vi "pid.vi"() -> (0 "Direct M3":bool, 1 "Pwm M3":dbl format="%#_13g", 2 "Pwm M2":dbl format="%#_13g", 3 "Pwm M1":dbl format="%#_13g", 4 "Direct M2":bool, 6 "Direct M1":bool, 9 "Counter Value 3":i32, 10 "Counter Value 2":i32, 11 "Counter Value":i32)   [LabVIEW 2015]
uses:
  <vilib>/myRIO/Common/Instrument Driver Framework/myRIO v1.0/Encoder/typedefs/Encoder Signal Mode.ctl
  <vilib>/myRIO/Instrument Drivers/Onboard IO/Encoder/typedefs/Encoder Reference.ctl
  <vilib>/myRIO/Common/Instrument Driver Framework/Utilities/typedefs/myRIO Generic Hardware Reference.ctl
  <vilib>/myRIO/Common/Instrument Driver Framework/Utilities/typedefs/Hardware Version Enum.ctl
  <vilib>/myRIO/Common/Instrument Driver Framework/Utilities/typedefs/myRIO v1.0 Reference.ctl
  <vilib>/myRIO/Common/Instrument Driver Framework/Utilities/typedefs/Generic FPGA Reference.ctl
  <vilib>/myRIO/Common/Instrument Driver Framework/myRIO v1.0/Encoder/typedefs/Encoder Channels Enum.ctl
  <vilib>/myRIO/Common/Instrument Driver Framework/myRIO v1.0/Encoder/typedefs/Encoder Configuration v1.0.ctl
  <vilib>/userdefined/High Color/nirio_resource_hc.ctl
  <vilib>/myRIO/Instrument Drivers/Onboard IO/DIO/typedefs/DIO Reference.ctl
  <vilib>/myRIO/Common/Instrument Driver Framework/myRIO v1.0/DIO/typedefs/DIO Channels List.ctl
  <vilib>/myRIO/Common/Instrument Driver Framework/myRIO v1.0/DIO/typedefs/DIO Channels Enum.ctl
  <vilib>/myRIO/Instrument Drivers/Onboard IO/PWM/typedefs/PWM Reference.ctl
  <vilib>/myRIO/Common/Instrument Driver Framework/myRIO v1.0/PWM/typedefs/PWM Channels Enum.ctl
  <vilib>/myRIO/Instrument Drivers/Onboard IO/PWM/typedefs/PWM Configuration.ctl
  <vilib>/myRIO/Common/Instrument Driver Framework/Utilities/vis/Is FPGA Ref Available.vi
  <vilib>/myRIO/Common/Instrument Driver Framework/myRIO v1.0/Encoder/vis/myRIO v1.1 Open Encoder.vi
  <vilib>/myRIO/Instrument Drivers/Onboard IO/Encoder/vis/Read.vi
  <vilib>/myRIO/Common/Instrument Driver Framework/myRIO v1.0/DIO/vis/myRIO v1.1 Open DIO.vi
  <vilib>/myRIO/Instrument Drivers/Onboard IO/DIO/vis/Write.vi
  <vilib>/myRIO/Common/Instrument Driver Framework/myRIO v1.0/PWM/vis/myRIO v1.1 Open PWM.vi
  <vilib>/myRIO/Instrument Drivers/Onboard IO/PWM/vis/Set Duty Cycle and Frequency.vi
  <vilib>/myRIO/Common/Instrument Driver Framework/Utilities/vis/Validate Channels.vi
  <vilib>/myRIO/Common/Instrument Driver Framework/myRIO v1.0/Encoder/vis/myRIO v1.0 Reserve Encoder.vi
  <vilib>/myRIO/Common/Instrument Driver Framework/myRIO v1.0/DIO/vis/myRIO v1.0 Reserve DIO.vi
  <vilib>/myRIO/Common/Instrument Driver Framework/myRIO v1.0/PWM/vis/myRIO v1.0 Reserve PWM.vi
  <vilib>/myRIO/Common/Instrument Driver Framework/myRIO v1.0/Encoder/vis/myRIO v1.0 Build MUX Configuration Encoder.vi
  <vilib>/myRIO/Common/Instrument Driver Framework/myRIO v1.0/Resource Manager/vis/myRIO v1.0 Reserve Channel List.vi
  <vilib>/myRIO/Common/Instrument Driver Framework/myRIO v1.0/DIO/vis/myRIO v1.0 Build MUX Configuration DIO.vi
  <vilib>/myRIO/Common/Instrument Driver Framework/myRIO v1.0/PWM/vis/myRIO v1.0 Build MUX Configuration PWM.vi
  <vilib>/myRIO/Common/Instrument Driver Framework/myRIO v1.0/Resource Manager/vis/myRIO v1.0 Create Configuration List.vi
  <vilib>/myRIO/Common/Instrument Driver Framework/myRIO v1.0/Resource Manager/vis/myRIO v1.0 Reserve Channel.vi
  <vilib>/myRIO/Common/Instrument Driver Framework/myRIO v1.0/Resource Manager/vis/myRIO v1.0 Unreserve Channel.vi
  <vilib>/myRIO/Common/Instrument Driver Framework/myRIO v1.0/Resource Manager/vis/myRIO v1.0 Build Mutex Name.vi
  <vilib>/Utility/VariantDataType/GetNumericInfo.vi
  <vilib>/Utility/error.llb/Error Cluster From Error Code.vi
  <vilib>/myRIO/Common/Instrument Driver Framework/myRIO v1.0/myRIO v1.1 Open.vi
  <vilib>/myRIO/Common/Instrument Driver Framework/Utilities/vis/IO Manager.vi
  <vilib>/myRIO/Common/Instrument Driver Framework/Utilities/vis/Configuration Manager.vi
  <vilib>/myRIO/Common/Instrument Driver Framework/myRIO v1.0/Resource Manager/vis/myRIO v1.0 Configure IO.vi
  <vilib>/myRIO/Common/Instrument Driver Framework/myRIO v1.0/myRIO v1.0 Close.vi
  <vilib>/myRIO/Common/Instrument Driver Framework/myRIO v1.0/Encoder/vis/myRIO v1.0 Configure Encoder.vi
  <vilib>/myRIO/Common/Instrument Driver Framework/myRIO v1.0/Encoder/vis/myRIO v1.0 Read Encoder.vi
  <vilib>/addons/control/pid/pid.llb/PID (DBL).vi
  <vilib>/myRIO/Common/Instrument Driver Framework/myRIO v1.0/DIO/vis/myRIO v1.0 Write DIO.vi
  <vilib>/myRIO/Common/Instrument Driver Framework/myRIO v1.0/PWM/vis/myRIO v1.0 Write PWM.vi
  <vilib>/myRIO/Express VI/Onboard IO/Encoder/Encoder Express VI.xnode
  <vilib>/myRIO/Instrument Drivers/Onboard IO/Encoder/vis/myRIO Encoder Open.xnode
  <vilib>/myRIO/Common/Instrument Driver Framework/myRIO v1.0/Encoder/typedefs/Encoder Count Direction Enum.ctl
  <vilib>/myRIO/Express VI/Onboard IO/DO/DO Express VI.xnode
  <vilib>/myRIO/Instrument Drivers/Onboard IO/DIO/vis/myRIO DIO Open.xnode
  <vilib>/myRIO/Express VI/Onboard IO/PWM/PWM Express VI.xnode
  <vilib>/myRIO/Instrument Drivers/Onboard IO/PWM/vis/myRIO PWM Open.xnode
  <vilib>/myRIO/Instrument Drivers/Onboard IO/Encoder/Encoder.lvlib
  <vilib>/addons/control/pid/NI_PID_pid.lvlib
  <vilib>/myRIO/Instrument Drivers/Onboard IO/DIO/DIO.lvlib
  <vilib>/myRIO/Instrument Drivers/Onboard IO/PWM/PWM.lvlib
panel:
  out "Waveform Chart 3":dynamicdata(graph)
  in  "PID gains 3":T1={"proportional gain (Kc)"=2.0, "integral time (Ti, min)"=0.001, "derivative time (Td, min)"=0.0} {"derivative time (Td, min)" format="%.3f"; "integral time (Ti, min)" format="%.3f"; "proportional gain (Kc)" format="%.3f"}
  out "output 3":dbl format="%.2f"
  in  "rpm 6":dbl(slide) scale=-230.0..230.0
  out "rpm 5":dbl
  out "Omega2 (rad/s) 3":dbl
  out "Omega(c/s) 3":dbl
  in  "Reset Counter 3":bool
  out "Waveform Chart 2":dynamicdata(graph)
  in  "PID gains 2":T1={"proportional gain (Kc)"=2.0, "integral time (Ti, min)"=0.001, "derivative time (Td, min)"=0.0} {"derivative time (Td, min)" format="%.3f"; "integral time (Ti, min)" format="%.3f"; "proportional gain (Kc)" format="%.3f"}
  out "output 2":dbl format="%.2f"
  in  "rpm 4":dbl(slide) scale=-230.0..230.0
  out "rpm 3":dbl
  out "Omega2 (rad/s) 2":dbl
  out "Omega(c/s) 2":dbl
  in  "Reset Counter 2":bool
  in  "stop":bool
  in  "Reset Counter":bool
  out "Omega(c/s)":dbl
  out "Omega2 (rad/s)":dbl
  out "rpm 2":dbl
  in  "rpm":dbl(slide) scale=-230.0..230.0
  out "output":dbl format="%.2f"
  in  "PID gains":T1={"proportional gain (Kc)"=2.0, "integral time (Ti, min)"=0.001, "derivative time (Td, min)"=0.0} {"derivative time (Td, min)" format="%.3f"; "integral time (Ti, min)" format="%.3f"; "proportional gain (Kc)" format="%.3f"}
  out "Waveform Chart":dynamicdata(graph)
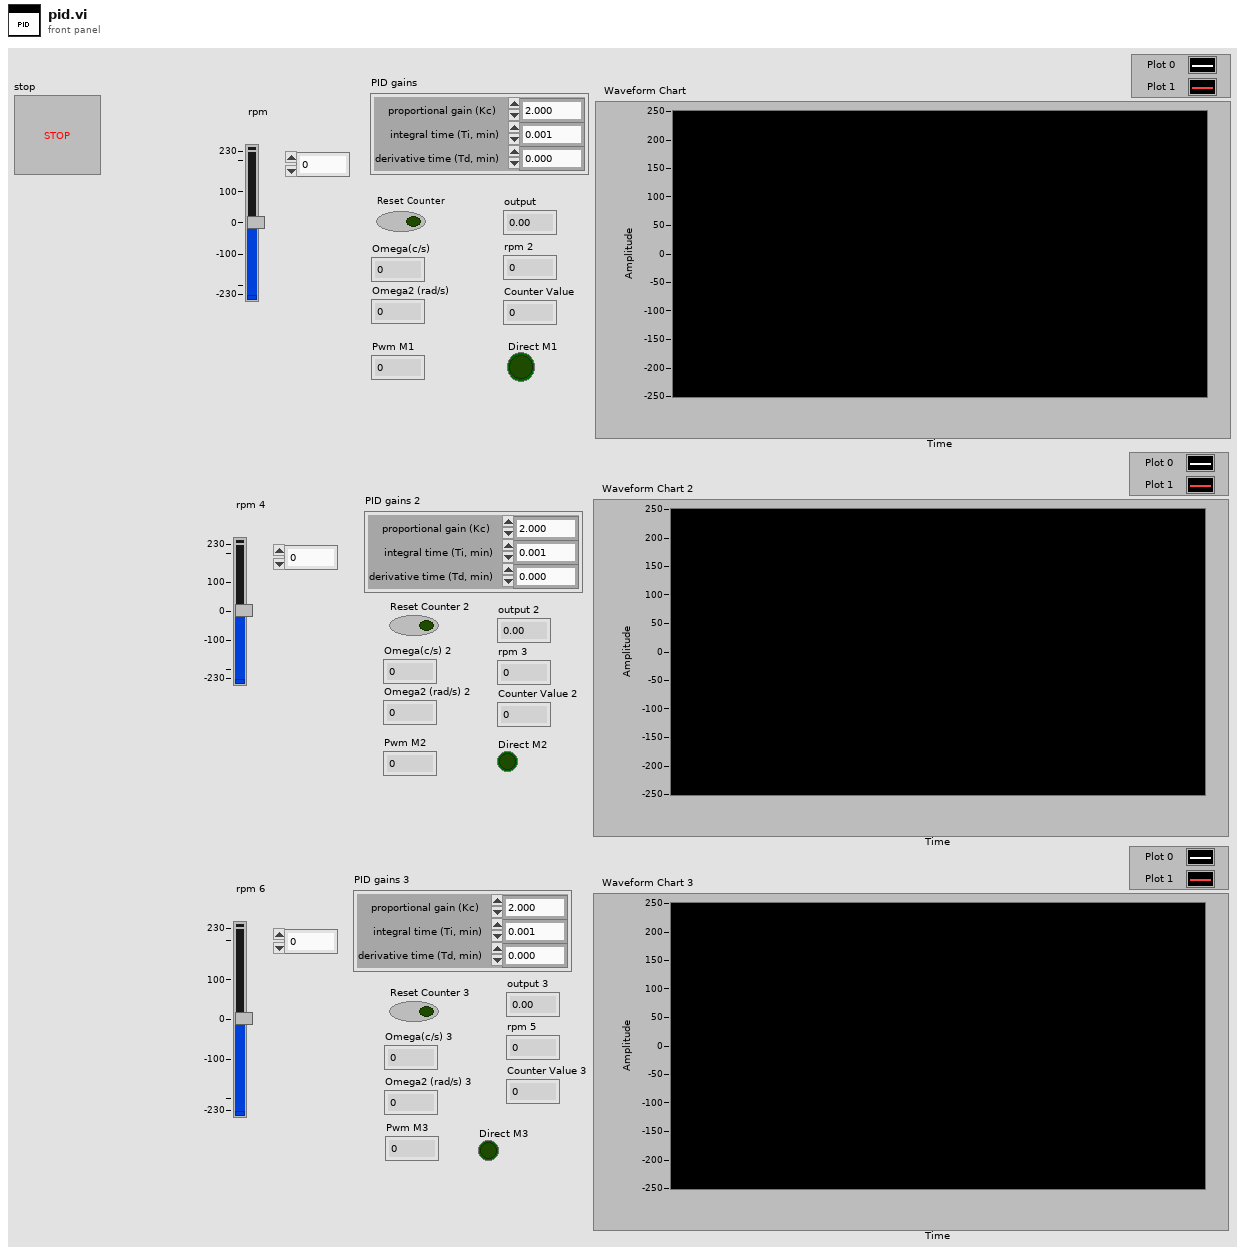
[diagram p1: front panel]
types:
  T1 = cluster{"proportional gain (Kc)":dbl, "integral time (Ti, min)":dbl, "derivative time (Td, min)":dbl}
  T2 = typedef "Encoder.lvlib/Encoder Reference.ctl" = cluster{"myRIO Reference":T3, "Encoder Channels Enum":T7}
  T3 = typedef "myRIO Generic Hardware Reference.ctl" = cluster{"myRIO Model":T4, "myRIO Hardware Reference":T5}
  T4 = typedef "Hardware Version Enum.ctl" = enum16{"Unknown", "myRIO-1900", "myRIO-1950", "roboRIO"}
  T5 = typedef "myRIO v1.0 Reference.ctl" = cluster{"Generic FPGA Reference":T6, "Allow multiple opens":bool}
  T6 = typedef "Generic FPGA Reference.ctl" = refnum<k20>
  T7 = typedef "Encoder Channels Enum.ctl" = enum16{"Not Connected", "C/ENC0", "C/ENC1", "A/ENC", "B/ENC", "DIO/ENC0", "DIO/ENC1", "DIO/ENC2", "DIO/ENC3", "DIO/ENC4"}
  T8 = typedef "Encoder Signal Mode.ctl" = enum16{"Quadrature phase signal", "Step and direction signal"}
  T9 = typedef "nirio_resource_hc.ctl" = tag
  T10 = typedef "PWM.lvlib/PWM Reference.ctl" = cluster{"myRIO Reference":T3, "PWM Channels Enum":T11, "PWM Configuration":T12}
  T11 = typedef "PWM Channels Enum.ctl" = enum16{"Not Connected", "C/PWM0", "C/PWM1", "A/PWM0", "A/PWM1", "A/PWM2", "B/PWM0", "B/PWM1", "B/PWM2", "PWM/PWM0", "PWM/PWM1", "PWM/PWM2", "PWM/PWM3", "PWM/PWM4", "PWM/PWM5", "PWM/PWM6", "PWM/PWM7", "PWM/PWM8", "PWM/PWM9"}
  T12 = typedef "PWM.lvlib/PWM Configuration.ctl" = cluster{"Frequency":dbl, "Duty Cycle":dbl}
  T13 = typedef "DIO.lvlib/DIO Reference.ctl" = cluster{"myRIO Reference":T3, "DIO Channels List":T14}
  T14 = typedef "DIO Channels List.ctl" = T15[]
  T15 = typedef "DIO Channels Enum.ctl" = enum16{"Not Connected", "C/DIO0", "C/DIO1", "C/DIO2", "C/DIO3", "C/DIO4", "C/DIO5", "C/DIO6", "C/DIO7", "A/DIO0", "A/DIO1", "A/DIO2", "A/DIO3", "A/DIO4", "A/DIO5", "A/DIO6", "A/DIO7", "A/DIO8", "A/DIO9", "A/DIO10", "A/DIO11", "A/DIO12", "A/DIO13", "A/DIO14", "A/DIO15", "B/DIO0", "B/DIO1", "B/DIO2", "B/DIO3", "B/DIO4", "B/DIO5", "B/DIO6", "B/DIO7", "B/DIO8", "B/DIO9", "B/DIO10", "B/DIO11", "B/DIO12", "B/DIO13", "B/DIO14", "B/DIO15", "LED0", "LED1", "LED2", "LED3", "Button0", "DIO/DIO0", "DIO/DIO1", "DIO/DIO2", "DIO/DIO3", "DIO/DIO4", "DIO/DIO5", "DIO/DIO6", "DIO/DIO7", "DIO/DIO8", "DIO/DIO9", "SPI/CS0", "SPI/CS1", "SPI/CS2", "SPI/CS3", "LED RADIO (Green)", "LED RADIO (Red)", "LED COMM (Green)", "LED COMM (Red)", "LED MODE (Green)", "LED MODE (Red)"}
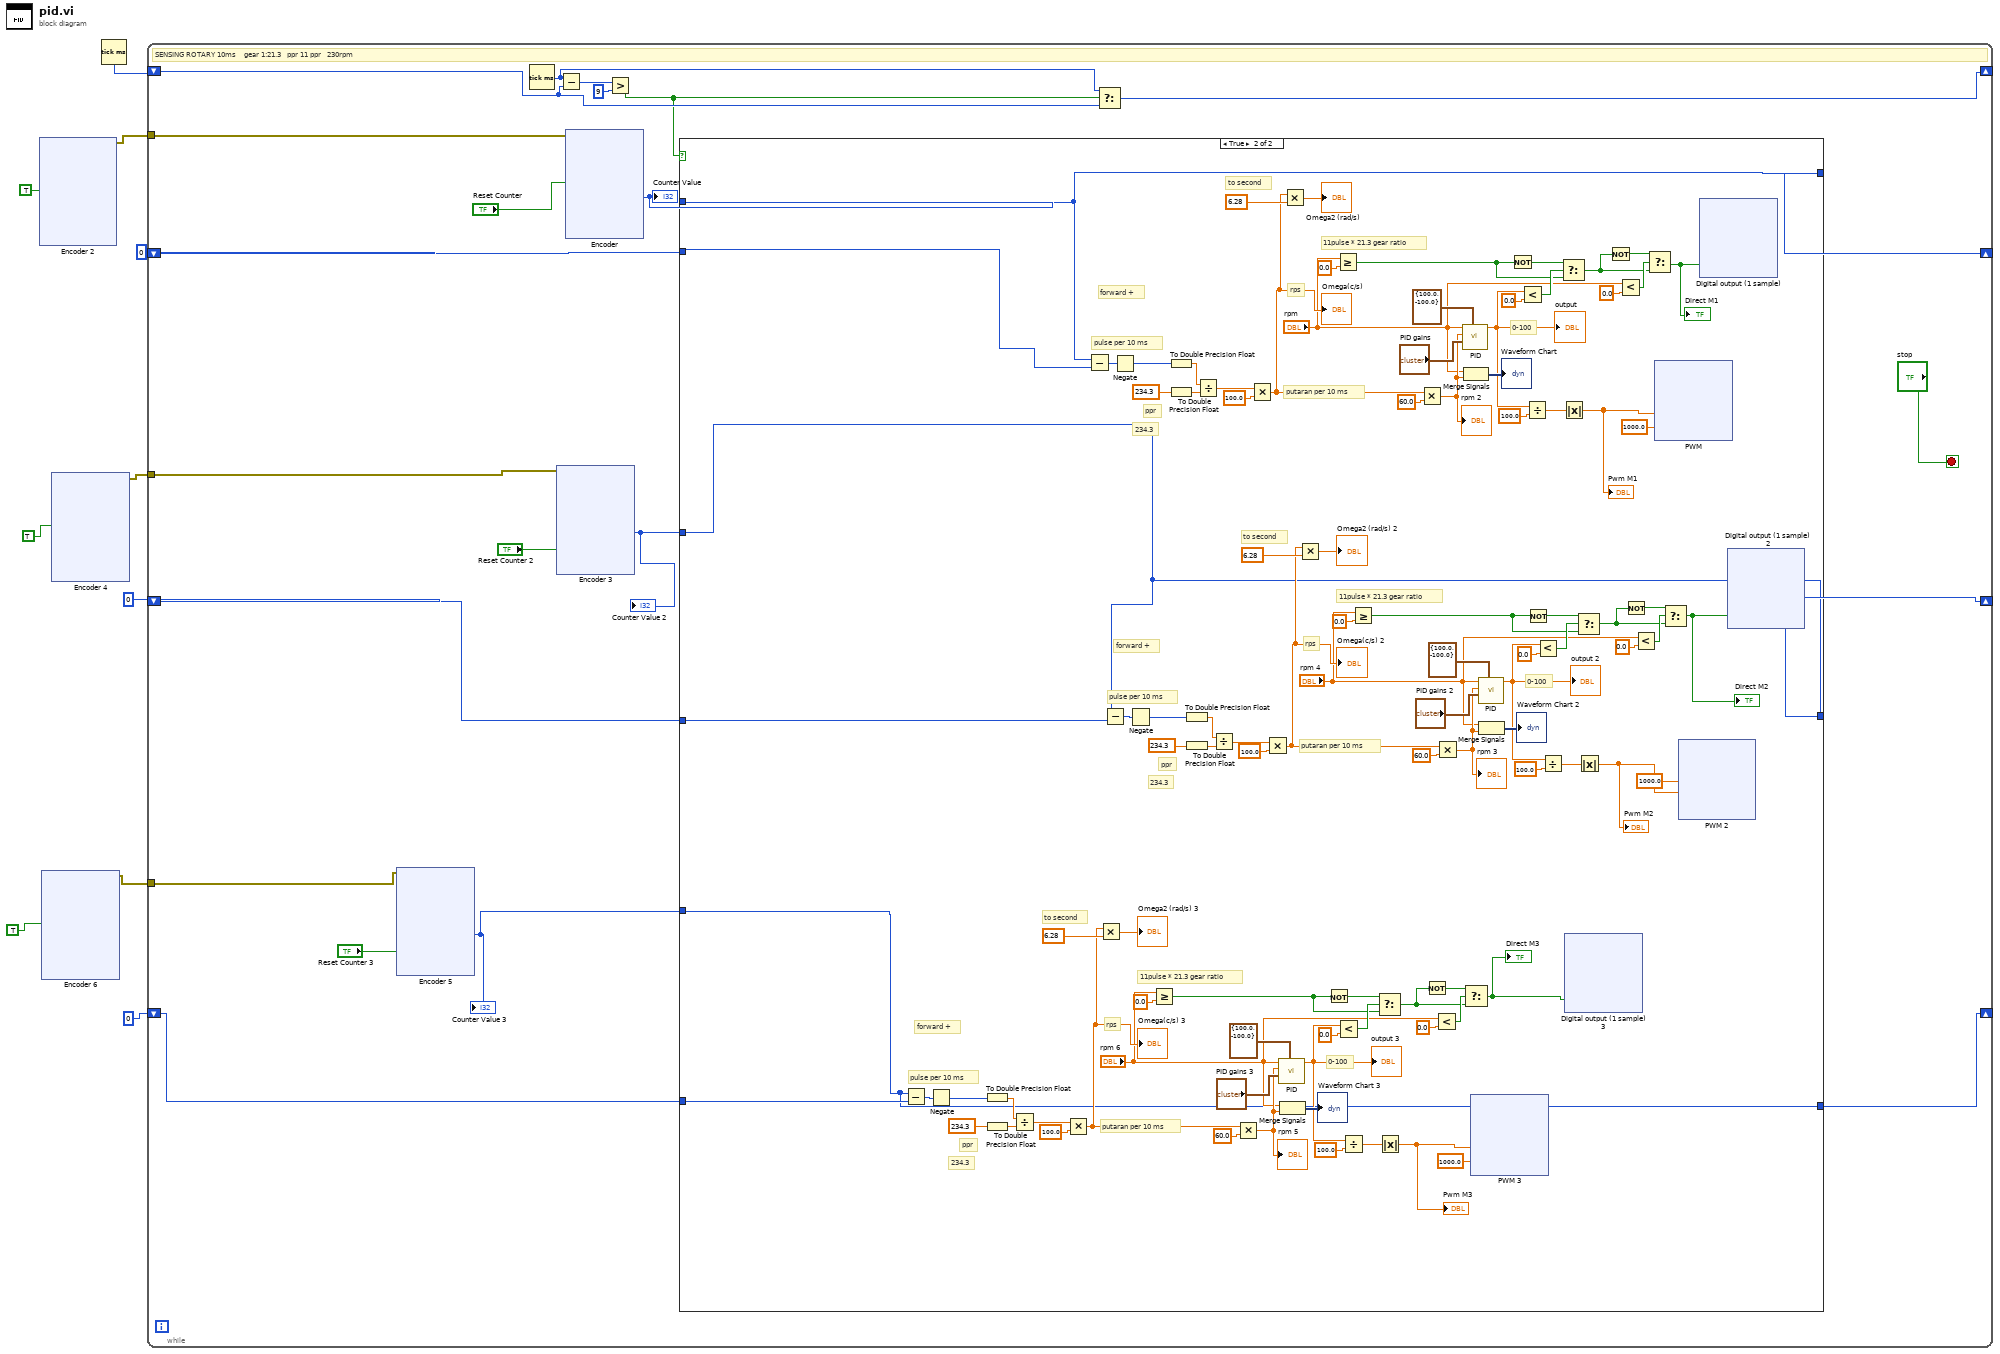
[diagram p0: block diagram]
diagram:
  n1 = xnode "Encoder 2"("Reset Counter"=TRUE) -> ("error out"=w9:errorcluster)  [unwired: 1 in, 3 out]
  n2 = xnode "Encoder 6"("Reset Counter"=TRUE) -> ("error out"=w4:errorcluster)  [unwired: 1 in, 3 out]
  n3 = xnode "Encoder 4"("Reset Counter"=TRUE) -> ("error out"=w7:errorcluster)  [unwired: 1 in, 3 out]
  n4 = Tick Count (ms)() -> (millisecond timer value=w10:u32)
  n5 = while {
    shift-right: [w28] -> _
    shift-left: w10 -> [w27]
    shift-right: [w22] -> _
    shift-left: 0 ("y") -> [w24]
    tunnel: w9 -> [w21]
    tunnel: w7 -> [w19]
    shift-right: [w16] -> _
    shift-left: 0 ("y") -> [w18]
    tunnel: w4 -> [w14]
    shift-right: [w11] -> _
    shift-left: 0 ("y") -> [w12]
    stop <- "stop" stop-if-true
    # "SENSING ROTARY 10ms    gear 1:21.3   ppr 11 ppr   230rpm"
    n6 = xnode "Encoder 5"("Reset Counter"="Reset Counter 3", "error in (no error)"=w14) -> ("Counter Value"=w13:i32)  [unwired: 3 out]
    "Counter Value 3" <- w13
    n7 = Tick Count (ms)() -> (millisecond timer value=w29:u32)
    n8 = xnode "Encoder 3"("Reset Counter"="Reset Counter 2", "error in (no error)"=w19) -> ("Counter Value"=w17:i32)  [unwired: 3 out]
    "Counter Value 2" <- w17
    n9 = Subtract(x=w29, y=w27) -> (x-y=w32:u32)
    n10 = xnode "Encoder"("Reset Counter"="Reset Counter", "error in (no error)"=w21) -> ("Counter Value"=w23:i32)  [unwired: 3 out]
    "Counter Value" <- w23
    n11 = Greater?(x=w32, y=u32 9) -> (0:w25:bool)
    n12 = case shown="True" w25 {
      tunnel: w24 -> [w127 w167]
      tunnel: w23 -> [_ w226]
      tunnel: [w127 w226] -> w22
      tunnel: w18 -> [w126 w166]
      tunnel: w17 -> [_ w165]
      tunnel: [w126 w165] -> w16
      tunnel: w13 -> [_ w134]
      tunnel: w12 -> [w125 w135]
      tunnel: [w125 w134] -> w11
      frame False {
      }
      frame True {
        # "rps"
        # "putaran per 10 ms"
        # "11pulse * 21.3 gear ratio"
        # "pulse per 10 ms"
        # "0-100"
        # "to second"
        # "ppr"
        # "234.3"
        # "forward +"
        # "rps"
        # "putaran per 10 ms"
        # "11pulse * 21.3 gear ratio"
        # "pulse per 10 ms"
        # "0-100"
        # "to second"
        # "ppr"
        # "234.3"
        # "forward +"
        # "rps"
        # "putaran per 10 ms"
        # "11pulse * 21.3 gear ratio"
        # "pulse per 10 ms"
        # "0-100"
        # "to second"
        # "ppr"
        # "234.3"
        # "forward +"
        n13 = Subtract(x=w134, y=w135) -> (x-y=w156:i32)
        n14 = Negate(x=w156) -> (-x=w164:i32)
        n15 = To Double Precision Float(number=w164) -> (double precision float=w161:dbl)
        n16 = To Double Precision Float(number=234.3) -> (double precision float=w159:dbl)
        n17 = Divide(x=w161, y=w159) -> (x/y=w158:dbl)
        n18 = Multiply(x=w158, y=100.0) -> (x*y=w154:dbl)
        "Omega(c/s) 3" <- w154
        n19 = Subtract(x=w226, y=w167) -> (x-y=w217:i32)
        n20 = Multiply(x=w154, y=6.28) -> (x*y=→"Omega2 (rad/s) 3":dbl)
        n21 = Subtract(x=w165, y=w166) -> (x-y=w188:i32)
        n22 = Negate(x=w217) -> (-x=w225:i32)
        n23 = Negate(x=w188) -> (-x=w196:i32)
        n24 = Greater Or Equal?(x="rpm 6", y=0.0) -> (x >= y?=w143:bool)
        n25 = To Double Precision Float(number=w225) -> (double precision float=w222:dbl)
        n26 = To Double Precision Float(number=234.3) -> (double precision float=w220:dbl)
        n27 = To Double Precision Float(number=w196) -> (double precision float=w193:dbl)
        n28 = To Double Precision Float(number=234.3) -> (double precision float=w191:dbl)
        n29 = Divide(x=w222, y=w220) -> (x/y=w219:dbl)
        n30 = Divide(x=w193, y=w191) -> (x/y=w190:dbl)
        n31 = Multiply(x=w154, y=60.0) -> (x*y=w150:dbl)
        "rpm 5" <- w150
        n32 = Multiply(x=w219, y=100.0) -> (x*y=w215:dbl)
        "Omega(c/s)" <- w215
        n33 = Multiply(x=w190, y=100.0) -> (x*y=w186:dbl)
        "Omega(c/s) 2" <- w186
        n34 = call-poly <vilib>:"PID.vi"("output range"=cluster{"output high":dbl, "output low":dbl} {"output high"=100.0, "output low"=-100.0}, "PID gains"="PID gains 3", "process variable"=w150, "setpoint"="rpm 6") -> ("output"=w148:dbl)  [unwired: 6 in, 1 out]
        "output 3" <- w148
        n35 = Merge Signals("rpm 6", w150) -> (→"Waveform Chart 3":dynamicdata)
        n36 = Multiply(x=w215, y=6.28) -> (x*y=→"Omega2 (rad/s)":dbl)
        n37 = Multiply(x=w186, y=6.28) -> (x*y=→"Omega2 (rad/s) 2":dbl)
        n38 = Not(x=w143) -> (.not. x?=w145:bool)
        n39 = Greater Or Equal?(x="rpm", y=0.0) -> (x >= y?=w204:bool)
        n40 = Less?(x=w148, y=0.0) -> (x < y?=w146:bool)
        n41 = Divide(x=w148, y=100.0) -> (x/y=w142:dbl)
        n42 = Greater Or Equal?(x="rpm 4", y=0.0) -> (x >= y?=w175:bool)
        n43 = Select(t=w145, s=w146, f=w143) -> (s? t:f=w137:bool)
        n44 = Absolute Value(x=w142) -> (abs(x)=w131:dbl)
        "Pwm M3" <- w131
        n45 = Multiply(x=w215, y=60.0) -> (x*y=w211:dbl)
        "rpm 2" <- w211
        n46 = Not(x=w137) -> (.not. x?=w138:bool)
        n47 = Less?(x="rpm 6", y=0.0) -> (x < y?=w141:bool)
        n48 = Multiply(x=w186, y=60.0) -> (x*y=w182:dbl)
        "rpm 3" <- w182
        n49 = call-poly <vilib>:"PID.vi"("output range"=cluster{"output high":dbl, "output low":dbl} {"output high"=100.0, "output low"=-100.0}, "PID gains"="PID gains", "process variable"=w211, "setpoint"="rpm") -> ("output"=w209:dbl)  [unwired: 6 in, 1 out]
        "output" <- w209
        n50 = Merge Signals("rpm", w211) -> (→"Waveform Chart":dynamicdata)
        n51 = Select(t=w138, s=w141, f=w137) -> (s? t:f=w128:bool)
        "Direct M3" <- w128
        n52 = xnode "PWM 3"("Duty Cycle"=w131, "Frequency [Hz]"=1000.0) -> ()  [unwired: 1 in, 1 out]
        n53 = call-poly <vilib>:"PID.vi"("output range"=cluster{"output high":dbl, "output low":dbl} {"output high"=100.0, "output low"=-100.0}, "PID gains"="PID gains 2", "process variable"=w182, "setpoint"="rpm 4") -> ("output"=w180:dbl)  [unwired: 6 in, 1 out]
        "output 2" <- w180
        n54 = Merge Signals("rpm 4", w182) -> (→"Waveform Chart 2":dynamicdata)
        n55 = Not(x=w204) -> (.not. x?=w206:bool)
        n56 = Less?(x=w209, y=0.0) -> (x < y?=w207:bool)
        n57 = Divide(x=w209, y=100.0) -> (x/y=w203:dbl)
        n58 = Not(x=w175) -> (.not. x?=w177:bool)
        n59 = Less?(x=w180, y=0.0) -> (x < y?=w178:bool)
        n60 = Divide(x=w180, y=100.0) -> (x/y=w174:dbl)
        n61 = Select(t=w206, s=w207, f=w204) -> (s? t:f=w198:bool)
        n62 = Absolute Value(x=w203) -> (abs(x)=w133:dbl)
        "Pwm M1" <- w133
        n63 = xnode "Digital output (1 sample) 3"("direction (B/DIO15 (Pin 34))"=w128) -> ()  [unwired: 1 in, 1 out]
        n64 = Select(t=w177, s=w178, f=w175) -> (s? t:f=w169:bool)
        n65 = Absolute Value(x=w174) -> (abs(x)=w132:dbl)
        "Pwm M2" <- w132
        n66 = Not(x=w198) -> (.not. x?=w199:bool)
        n67 = Less?(x="rpm", y=0.0) -> (x < y?=w202:bool)
        n68 = Not(x=w169) -> (.not. x?=w170:bool)
        n69 = Less?(x="rpm 4", y=0.0) -> (x < y?=w173:bool)
        n70 = Select(t=w199, s=w202, f=w198) -> (s? t:f=w129:bool)
        "Direct M1" <- w129
        n71 = xnode "PWM"("Duty Cycle"=w133, "Frequency [Hz]"=1000.0) -> ()  [unwired: 1 in, 1 out]
        n72 = Select(t=w170, s=w173, f=w169) -> (s? t:f=w130:bool)
        "Direct M2" <- w130
        n73 = xnode "PWM 2"("Duty Cycle"=w132, "Frequency [Hz]"=1000.0) -> ()  [unwired: 1 in, 1 out]
        n74 = xnode "Digital output (1 sample)"("direction (B/DIO13 (Pin 26))"=w129) -> ()  [unwired: 1 in, 1 out]
        n75 = xnode "Digital output (1 sample) 2"("direction (B/DIO14 (Pin 32))"=w130) -> ()  [unwired: 1 in, 1 out]
      }
    }
    n76 = Select(t=w29, s=w25, f=w27) -> (s? t:f=w28:u32)
  }
